vi "CloseMetodo.vi"(8 "error in (no error)":errorcluster, 11 "TektroniksTDS in":refnum<class "TektroniksTDS.lvclass">) -> (0 "error out":errorcluster, 3 "TektroniksTDS out":refnum<class "TektroniksTDS.lvclass">)   [LabVIEW 2020, in "TektroniksTDS.lvclass"]
uses:
  TektroniksTDS.lvclass
  TektroniksTDS.lvclass/TektroniksTDS.ctl
  Osciloscope/Osciloscope.lvclass
  <instrlib>/Tektronix TDS 200 1000 2000 Series/Tektronix TDS 200 1000 2000 Series.lvlib
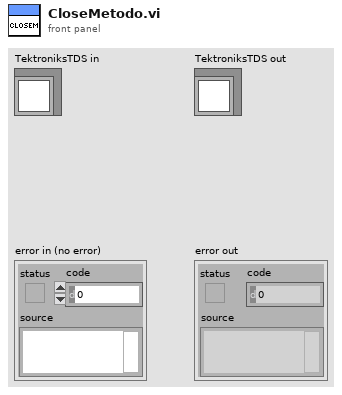
[diagram p1: front panel]
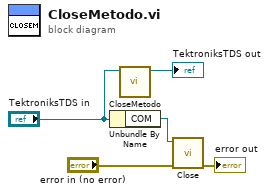
[diagram p0: block diagram]
diagram:
  n1 = Unbundle By Name("TektroniksTDS in") -> ("COM"=w3:refnum<visa-resource-name>)
  n2 = call-parent "CloseMetodo.vi"("Osciloscope in"="TektroniksTDS in") -> ("Osciloscope out"=→"TektroniksTDS out":refnum<class "TektroniksTDS.lvclass">)  [unwired: 9 in, 1 out]
  n3 = call <instrlib>:"Close.vi"("error in (no error)"="error in (no error)", "VISA resource name"=w3) -> ("error out"=→"error out":errorcluster)  [unwired: 9 in]
